vi "Write Ref.vi"(8 "error in (no error)":errorcluster, 10 "config data":T1, 11 "Config Data in":refnum<class "Config Data.lvclass">) -> (0 "error out":errorcluster, 3 "Config Data out":refnum<class "Config Data.lvclass">)   [LabVIEW 2018, in "Config Data.lvclass"]
uses:
  Config Data.lvclass
  <vilib>/Utility/config.llb/Config Data RefNum.ctl
  Config Data.lvclass/Config Data.ctl
  <vilib>/Utility/config.llb/NI_LVConfig.lvlib
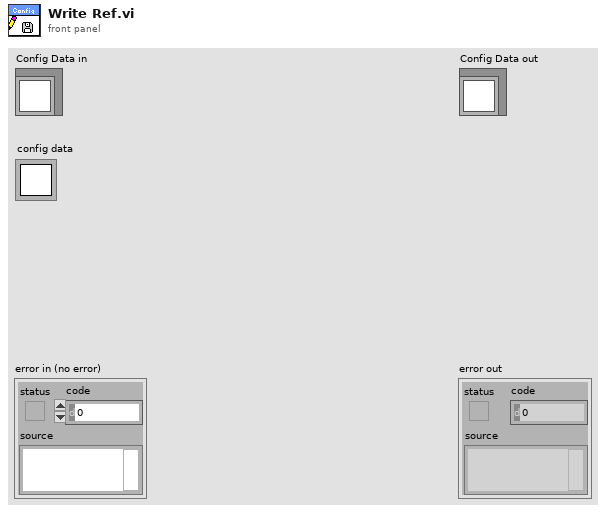
[diagram p1: front panel]
types:
  T1 = typedef "NI_LVConfig.lvlib/Config Data RefNum.ctl" = refnum<k1>
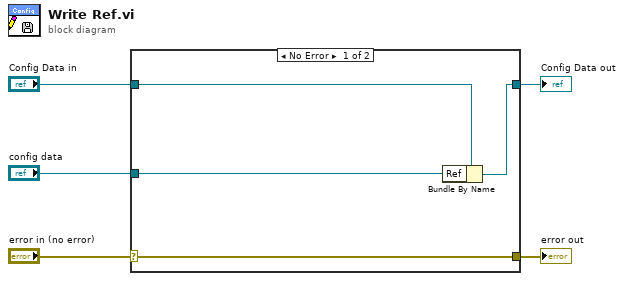
[diagram p0: block diagram]
diagram:
  n1 = case shown="No Error" "error in (no error)" {
    selector: "error in (no error)" -> [w9 w10]
    tunnel: [w9 w10] -> w4
    tunnel: [w7 w11] -> w2
    tunnel: "Config Data in" -> [w8 w11]
    tunnel: "config data" -> [w6 _]
    frame No Error {
      n2 = Bundle By Name(cluster=w8, "Ref"=w6) -> (w7:refnum<class "Config Data.lvclass">)
    }
    frame Error {
    }
  }
  "error out" <- w4
  "Config Data out" <- w2
